vi "display fits.vi"(0 "LineCCD in":refnum<class "LineCCD.lvclass">, 5 "error in (no error)":errorcluster) -> (12 "LPA":cluster{cdb[]}[](graph), 14 "LineCCD out":refnum<class "LineCCD.lvclass">, 15 "LPB":cluster{cdb[]}[](graph), 18 "Line profile":cluster{cdb[]}[](graph), 19 "error out":errorcluster)   [LabVIEW 2012, in "LineCCD.lvclass"]
uses:
  LineCCD.lvclass
  LineCCD.lvclass/LineCCD.ctl
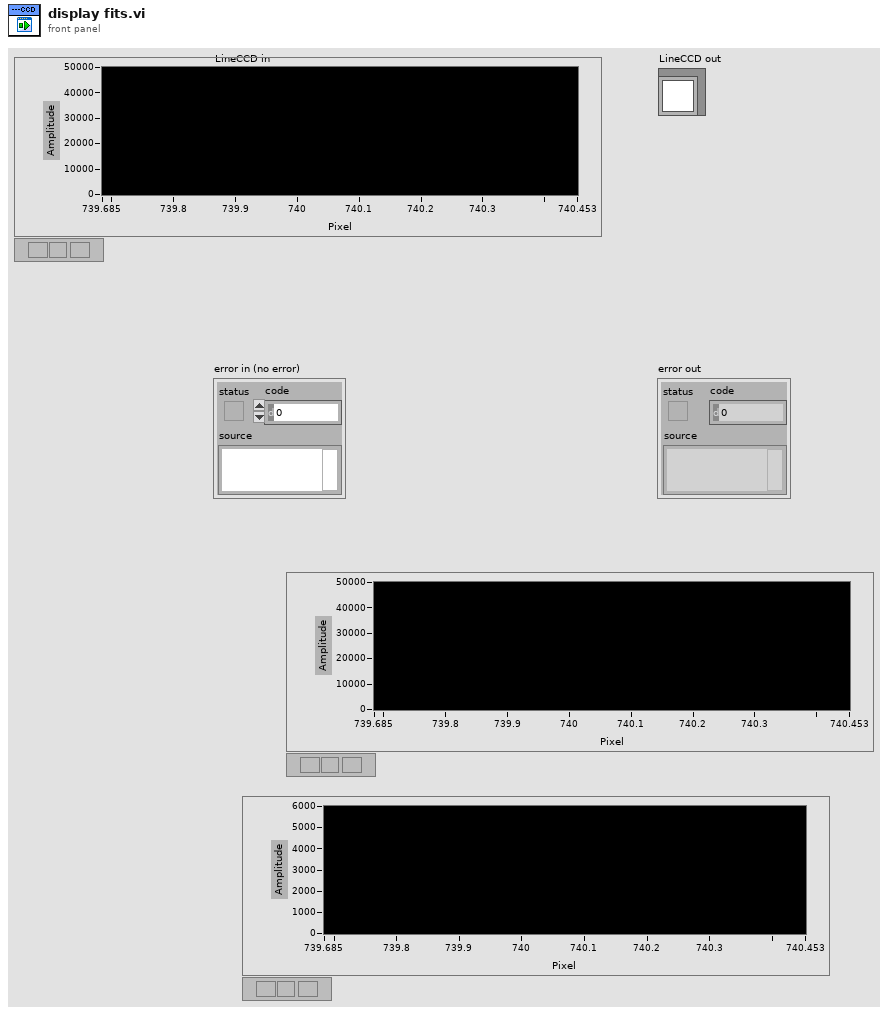
[diagram p1: front panel]
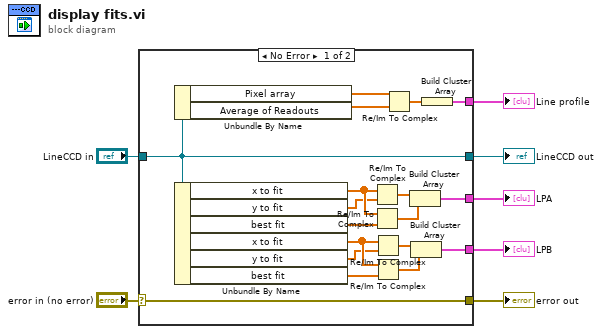
[diagram p0: block diagram]
diagram:
  n1 = case shown="No Error" "error in (no error)" {
    selector: "error in (no error)" -> [w25 w27]
    tunnel: [w25 w27] -> w6
    tunnel: [w12 w26] -> w4
    tunnel: "LineCCD in" -> [w12 w26]
    tunnel: [w19 _] -> w3
    tunnel: [w13 _] -> w2
    tunnel: [w8 _] -> w1
    frame No Error {
      n2 = Unbundle By Name(w12) -> ("Pixel array"=w10:dbl[], "Average of Readouts"=w9:dbl[])
      n3 = Unbundle By Name(w12) -> ("x to fit"=w23:dbl[], "y to fit"=w22:dbl[], "best fit"=w21:dbl[], "x to fit"=w16:dbl[], "y to fit"=w15:dbl[], "best fit"=w14:dbl[])
      n4 = Re/Im To Complex(1:w22, 2:w23) -> (0:w20:cdb[])
      n5 = Re/Im To Complex(1:w21, 2:w23) -> (0:w24:cdb[])
      n6 = Re/Im To Complex(1:w15, 2:w16) -> (0:w18:cdb[])
      n7 = Re/Im To Complex(1:w14, 2:w16) -> (0:w17:cdb[])
      n8 = Re/Im To Complex(1:w9, 2:w10) -> (0:w11:cdb[])
      n9 = Build Cluster Array(w20, w24) -> (w19:cluster{cdb[]}[])
      n10 = Build Cluster Array(w18, w17) -> (w13:cluster{cdb[]}[])
      n11 = Build Cluster Array(w11) -> (w8:cluster{cdb[]}[])
    }
    frame Error {
    }
  }
  "error out" <- w6
  "LineCCD out" <- w4
  "LPA" <- w3
  "LPB" <- w2
  "Line profile" <- w1
